vi "Game Engine.vi"(6 "UI Refs":T1, 8 "XY":cluster{"Horizontal":dbl, "Vertical":dbl}, 10 "Dashboard":T2[](array[typedef]), 11 "SquareBattle in":refnum<class "SquareBattle Arena.lvclass">) -> ()   [LabVIEW 2014, in "SquareBattle Arena.lvlib" / "SquareBattle Arena.lvclass"]
uses:
  SquareBattle Arena.lvclass
  Dashboard.ctl
  UI Refs.ctl
  Runner Cluster.ctl
  Square/Square.lvclass
  SquareBattle Arena.lvclass/SquareBattle Arena.ctl
  Action Enum.ctl
  Square/Square.lvclass/Square.ctl
  Endigit Library/Endigit.lvlib
panel:
  out "Penalty":i32(graph)
  out "Total Runners":i32
  out "Elapsed Time":u32
  # "NOTICE - YOU MUST NOT REMOVE THIS NOTICE. PER THE FOLLOWING LICENSE, YOU MAY REPRODUCE THIS SOFTWARE PROVIDED YOU FOLLOW THE TERMS\nOF THE LICENSE.\n\n---BEGIN BSD LICENSE (http://opensource.org/licenses/BSD-2-Clause)---\nCopyright (c) 2015, Endigit, Inc. <robert@endigit.com>\nAll rights reserved.\n\nRedistribution and use in source and binary forms, with or without modification, are permitted provided that the following conditions are met:\n\n1. Redistributions of source code must retain the above copyright notice, this list of conditions and the following disclaimer.\n\n2. Redistributions in binary form must reproduce the above copyright notice, this list of conditions and the following disclaimer in the documentation and/or other \nmaterials provided with the distribution.\n\nTHIS SOFTWARE IS PROVIDED BY THE COPYRIGHT HOLDERS AND CONTRIBUTORS \"AS IS\" AND ANY EXPRESS OR IMPLIED WARRANTIES, INCLUDING, BUT NOT \nLIMITED TO, THE IMPLIED WARRANTIES OF MERCHANTABILITY AND FITNESS FOR A PARTICULAR PURPOSE ARE DISCLAIMED. IN NO EVENT SHALL THE COPYRIGHT \nHOLDER OR CONTRIBUTORS BE LIABLE FOR ANY DIRECT, INDIRECT, INCIDENTAL, SPECIAL, EXEMPLARY, OR CONSEQUENTIAL DAMAGES (INCLUDING, BUT NOT \nLIMITED TO, PROCUREMENT OF SUBSTITUTE GOODS OR SERVICES; LOSS OF USE, DATA, OR PROFITS; OR BUSINESS INTERRUPTION) HOWEVER CAUSED AND ON \nANY THEORY OF LIABILITY, WHETHER IN CONTRACT, STRICT LIABILITY, OR TORT (INCLUDING NEGLIGENCE OR OTHERWISE) ARISING IN ANY WAY OUT OF THE USE \nOF THIS SOFTWARE, EVEN IF ADVISED OF THE POSSIBILITY OF SUCH DAMAGE.\n---END BSD LICENSE---"
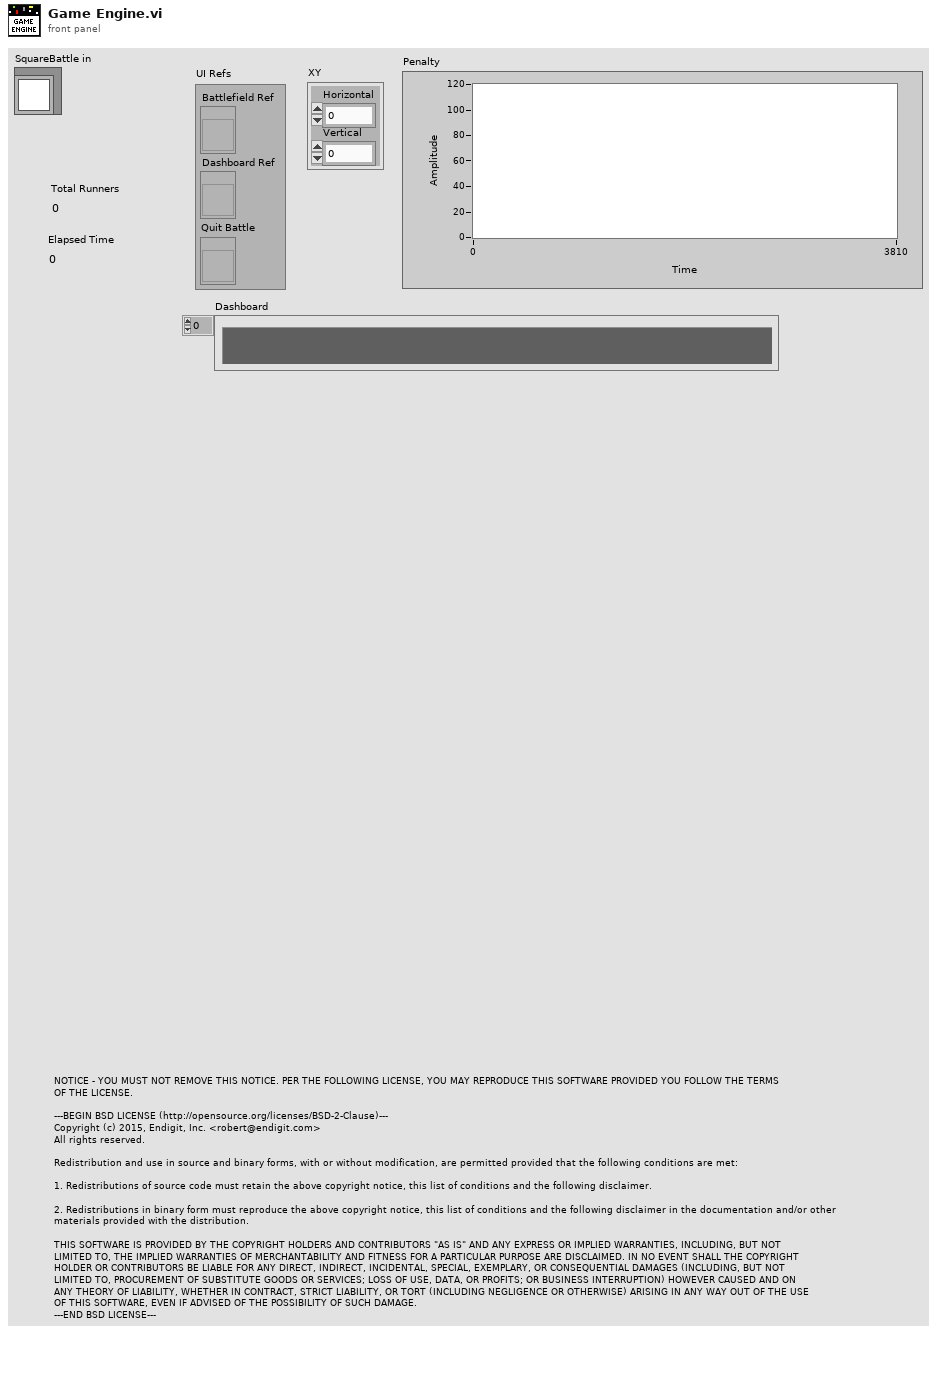
[diagram p1: front panel]
types:
  T1 = typedef "SquareBattle Arena.lvlib/SquareBattle Arena.lvclass/UI Refs.ctl" = cluster{"Battlefield Ref":refnum<vi>, "Dashboard Ref":refnum<vi>, "Quit Battle":refnum<vi>}
  T2 = typedef "SquareBattle Arena.lvlib/SquareBattle Arena.lvclass/Dashboard.ctl" = cluster{"Color":u32, "Player":string, "Status":string}
  T3 = typedef "SquareBattle Arena.lvlib/SquareBattle Arena.lvclass/Runner Cluster.ctl" = cluster{"Attacked?":bool, "DVR":refnum<data-value>, "Team":i32, "Player":i32, "Next Turn":i32, "Penalty":i32}
  T4 = typedef "SquareBattle Arena.lvlib/SquareBattle Arena.lvclass/Action Enum.ctl" = enum16{"Wait", "Move", "Attack", "Replicate"}
  T5 = typedef "SquareBattle Arena.lvlib/SquareBattle Arena.lvclass/Direction Enum.ctl" = enum16{"NW", "N", "NE", "E", "SE", "S", "SW", "W"}
  T6 = cluster{"Cluster":T3, i32, i32, "Action":T4, "Direction":T5, "Replicated":refnum<class "Square.lvclass">}
  T7 = typedef "SquareBattle Arena.lvlib/SquareBattle Arena.lvclass/Player Info.ctl" = cluster{"Name":string, "Color Box":u32, "Gloat Phrase":string}
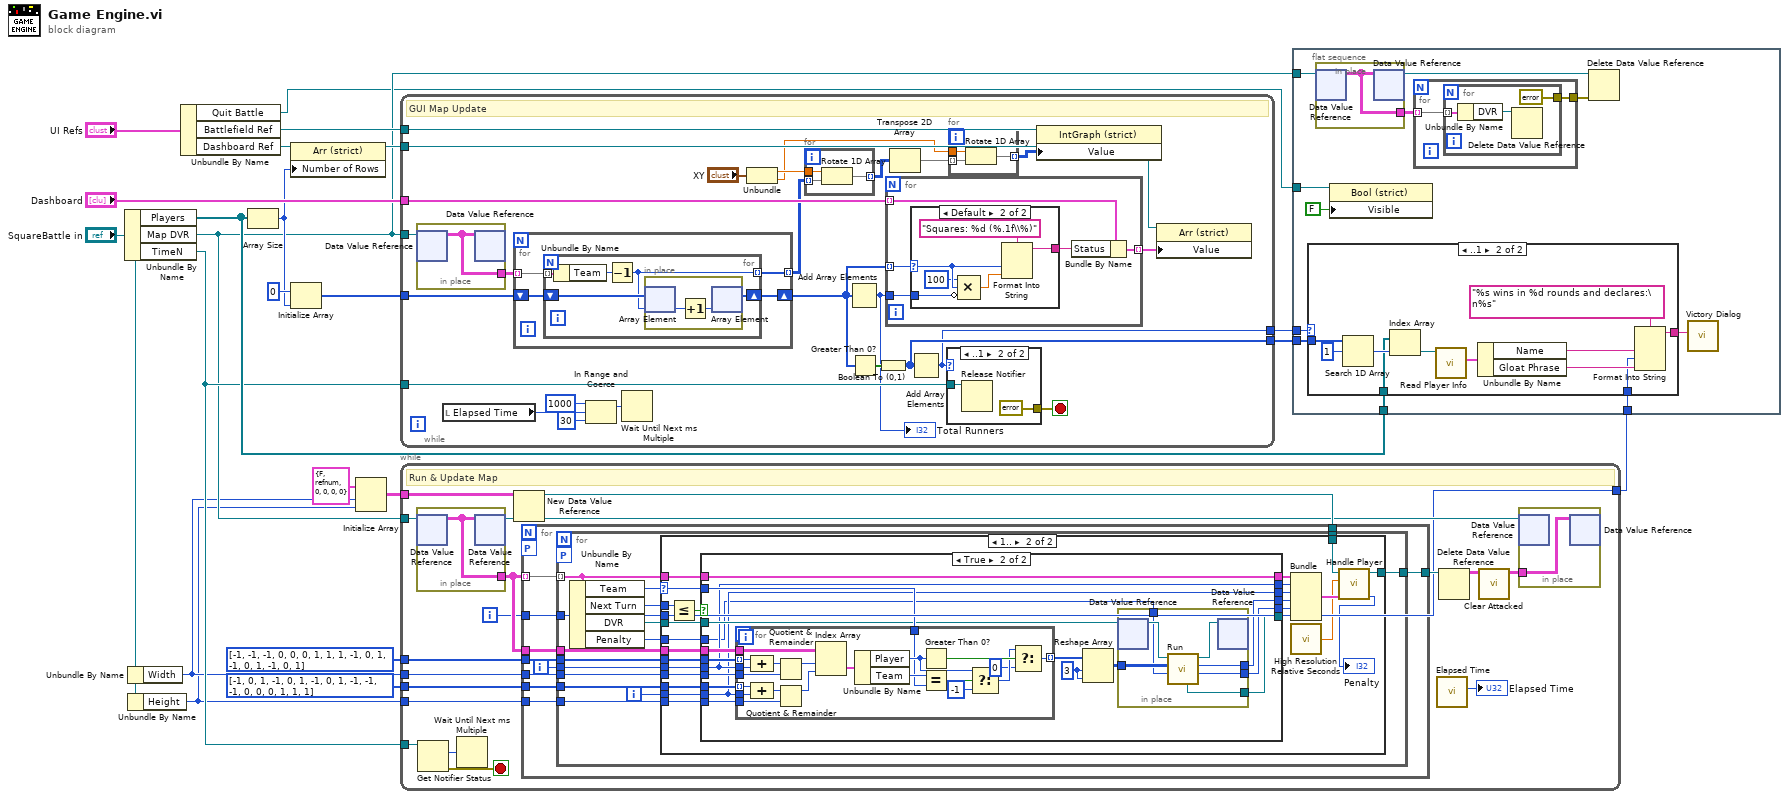
[diagram p0: block diagram]
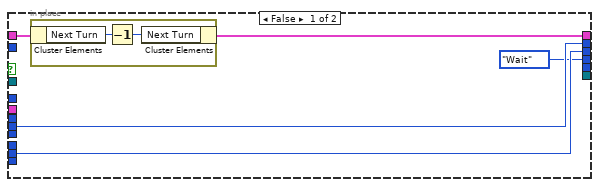
[diagram p3: hidden frame]
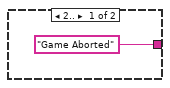
[diagram p4: hidden frame]
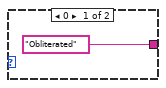
[diagram p5: hidden frame]
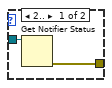
[diagram p6: hidden frame]
diagram:
  n1 = Unbundle By Name("SquareBattle in") -> ("Players"=w12:refnum<class "Square.lvclass">[], "Map DVR"=w10:refnum<data-value>, "TimeN"=w11:refnum<notifier>)
  n2 = Unbundle By Name("SquareBattle in") -> ("Width"=w7:i32)
  n3 = Unbundle By Name("SquareBattle in") -> ("Height"=w6:i32)
  n4 = Unbundle By Name("UI Refs") -> ("Quit Battle"=w4:refnum<vi>, "Battlefield Ref"=w20:refnum<vi>, "Dashboard Ref"=w17:refnum<vi>)
  n5 = Array Size(array=w12) -> (size(s)=w14:i32)
  n6 = property on="Property Node" class="Arr (strict)"(reference=w17, "Number of Rows"=w14) -> (reference out=w16:refnum<vi>)  [unwired: 1 in, 1 out]
  n7 = Initialize Array(0 ("element"), w14) -> (w13:i32[])
  n8 = Initialize Array(T3 {"Attacked?"=FALSE, "DVR"=refnum, "Team"=0, "Player"=0, "Next Turn"=0, "Penalty"=0} ("Cluster"), w7, w6) -> (w5:T3[][])
  n9 = while {
    tunnel: "Dashboard" -> [w45]
    tunnel: w16 -> [w42]
    tunnel: w20 -> [w26]
    tunnel: [w34] -> w19
    tunnel: [w33] -> w18
    tunnel: w10 -> [w36]
    tunnel: w11 -> [w38]
    tunnel: w13 -> [w37]
    stop <- w46 stop-if-true
    # "GUI Map Update"
    n10 = in-place {
      in-place-border: [w65] -> w35
      n11 = in-place-dvr #1(w36) -> (w65:T3[][])  [unwired: 1 out]
      n12 = in-place-dvr #1(w65) -> ()  [unwired: 2 out]
    }
    n13 = local read "Elapsed Time"() -> (w31:u32)
    n14 = for {
      tunnel: w35 -> [w55] mode=indexing
      tunnel: [w54] -> w30 mode=indexing
      shift-right: [w57] -> w44
      shift-left: w37 -> [w56]
      n15 = for {
        shift-right: [w62] -> w57
        shift-left: w56 -> [w61]
        tunnel: w55 -> [w60] mode=indexing
        tunnel: [w58] -> w54 mode=indexing
        n16 = Unbundle By Name(w60) -> ("Team"=w59:i32)
        n17 = Decrement(x=w59) -> (x-1=w58:i32)
        n18 = in-place {
          n19 = in-place-array #2(w61, w58) -> (w64:i32)
          n20 = Increment(x=w64) -> (x+1=w63:i32)
          n21 = in-place-array #2(w63) -> (w62:i32[])  [unwired: 1 out]
        }
      }
    }
    n22 = In Range and Coerce(upper limit=u32 1000 ("millisecond multiple"), x=w31, lower limit=u32 30) -> (coerced(x)=w41:u32)  [unwired: 1 out]
    n23 = Wait Until Next ms Multiple(millisecond multiple=w41) -> ()  [unwired: 1 out]
    n24 = Unbundle("XY") -> ("Horizontal"=w24:dbl, "Vertical"=w23:dbl)
    n25 = for {
      tunnel: w30 -> [w53] mode=indexing
      tunnel: [w52] -> w29 mode=indexing
      tunnel: w24 -> [w51]
      n26 = Rotate 1D Array(1:w53, 2:w51) -> (0:w52:i32[])
    }
    n27 = Add Array Elements(numeric array=w44) -> (sum=w32:i32)
    "Total Runners" <- w32
    n28 = Greater Than 0?(x=w44) -> (x > 0?=w47:bool[])
    n29 = Boolean To (0,1)(Boolean=w47) -> (0, 1=w34:i16[])
    n30 = for {
      tunnel: w45 -> [w70] mode=indexing
      tunnel: [w69] -> w43 mode=indexing
      tunnel: w44 -> [w66] mode=indexing
      tunnel: w32 -> [w67]
      n31 = case shown="Default" w66 {
        selector: w66 -> [_ w74]
        tunnel: ["Obliterated" w76] -> w68
        tunnel: w67 -> [_ w73]
        frame 0 {
        }
        frame Default {
          n32 = Compound Arithmetic op=MULTIPLY(100 ("value"), w74, invert w73) -> (w75:dbl)
          n33 = Format Into String(format string="Squares: %d (%.1f\\%)", w74, w75) -> (resulting string=w76:string)  [unwired: 2 in, 1 out]
        }
      }
      n34 = Bundle By Name(cluster=w70, "Status"=w68) -> (w69:T2)
    }
    n35 = Transpose 2D Array(2D array=w29) -> (transposed array=w28:i32[][])
    n36 = Add Array Elements(numeric array=w34) -> (sum=w33:i16)
    n37 = case shown="..1" w33 {
      tunnel: w38 -> [w79 w81]
      tunnel: [w78 errorcluster {"status"=TRUE, "code"=0, "source"=""} ("error out")] -> w46
      frame 2.. {
        n38 = Get Notifier Status(notifier=w79) -> (error out=w78:errorcluster)  [unwired: 1 in, 4 out]
      }
      frame ..1 {
        n39 = Release Notifier(notifier=w81) -> ()  [unwired: 2 in, 3 out]
      }
    }
    n40 = for {
      tunnel: w28 -> [w50] mode=indexing
      tunnel: [w49] -> w27 mode=indexing
      tunnel: w23 -> [w48]
      n41 = Rotate 1D Array(1:w50, 2:w48) -> (0:w49:i32[])
    }
    n42 = property on="Property Node" class="IntGraph (strict)"(reference=w26, "Value"=w27) -> ()  [unwired: 1 in, 2 out]
    n43 = property on="Property Node" class="Arr (strict)"(reference=w42, "Value"=w43) -> ()  [unwired: 1 in, 2 out]
  }
  n44 = while {
    tunnel: w11 -> [w97]
    tunnel: w10 -> [w95]
    tunnel: i32[] [-1, -1, -1, 0, 0, 0, 1, 1, 1, -1, 0, 1, -1, 0, 1, -1, 0, 1] -> [w93]
    tunnel: w7 -> [w92]
    tunnel: i32[] [-1, 0, 1, -1, 0, 1, -1, 0, 1, -1, -1, -1, 0, 0, 0, 1, 1, 1] -> [w90]
    tunnel: w6 -> [w91]
    tunnel: w5 -> [w89]
    tunnel: [w82] -> w1
    i -> [w82]
    stop <- w96 stop-if-true
    # "Run & Update Map"
    n45 = in-place {
      in-place-border: [w203] -> w94
      n46 = in-place-dvr #3(w95) -> (w203:T3[][])  [unwired: 1 out]
      n47 = in-place-dvr #3(w203) -> (w86:refnum<data-value>)  [unwired: 1 out]
    }
    n48 = Get Notifier Status(notifier=w97) -> (current notification=w98:u32, error out=w96:errorcluster)  [unwired: 1 in, 3 out]
    n49 = Wait Until Next ms Multiple(millisecond multiple=w98) -> ()  [unwired: 1 out]
    n50 = New Data Value Reference(data value=w89) -> (data value reference=w88:refnum<data-value>)  [unwired: 1 in, 1 out]
    n51 = for {
      tunnel: w94 -> [w109] mode=indexing
      tunnel: w82 -> [w108]
      tunnel: w94 -> [w107]
      tunnel: w93 -> [w106]
      tunnel: w92 -> [w104]
      tunnel: w90 -> [w102]
      tunnel: w91 -> [w103]
      tunnel: w88 -> [w101]
      tunnel: [w100] -> w87
      workers-P: _ -> [_]
      i -> [w105]
      n52 = for {
        tunnel: w109 -> [w115] mode=indexing
        tunnel: w108 -> [w114]
        tunnel: w107 -> [w124]
        tunnel: w106 -> [w123]
        tunnel: w105 -> [w122]
        tunnel: w104 -> [w121]
        tunnel: w102 -> [w119]
        tunnel: w103 -> [w120]
        workers-P: _ -> [_]
        tunnel: w101 -> [w112]
        tunnel: [w111] -> w100
        i -> [w118]
        n53 = Unbundle By Name(w115) -> ("Team"=w116:i32, "Next Turn"=w113:i32, "DVR"=w117:refnum<data-value>, "Penalty"=w110:i32)
        n54 = case shown="1.." w116 {
          selector: w116 -> [_ w145]
          tunnel: w124 -> [_ w150]
          tunnel: w123 -> [_ w149]
          tunnel: w122 -> [_ w142]
          tunnel: w121 -> [_ w148]
          tunnel: w119 -> [_ w146]
          tunnel: w118 -> [_ w141]
          tunnel: w120 -> [_ w147]
          tunnel: w117 -> [_ w144]
          tunnel: w115 -> [_ w143]
          tunnel: w114 -> [_ w140]
          tunnel: w113 -> [_ w139]
          tunnel: w112 -> [w125 w130]
          tunnel: [w125 w129] -> w111
          tunnel: w110 -> [_ w126]
          frame ..0 {
          }
          frame 1.. {
            n55 = Less Or Equal?(x=w139, y=w140) -> (x <= y?=w138:bool)
            n56 = case shown="True" w138 {
              tunnel: w150 -> [_ w174]
              tunnel: w149 -> [_ w173]
              tunnel: w148 -> [_ w172]
              tunnel: w147 -> [_ w171]
              tunnel: w146 -> [_ w170]
              tunnel: w145 -> [_ w167]
              tunnel: w144 -> [_ w165]
              tunnel: w143 -> [w152 w164]
              tunnel: w142 -> [w155 w163]
              tunnel: w141 -> [w154 w162]
              tunnel: [w151 w164] -> w137
              tunnel: [w155 w163] -> w136
              tunnel: [w154 w162] -> w135
              tunnel: [Action_Enum."Wait" ("Action") w161] -> w134
              tunnel: [_ w160] -> w133
              tunnel: [_ w159] -> w132
              tunnel: w126 -> [_ w158]
              frame False {
                n57 = in-place {
                  n58 = in-place-cluster #4(w152) -> ("Next Turn"=w157:i32)
                  n59 = Decrement(x=w157) -> (x-1=w156:i32)
                  n60 = in-place-cluster #4("Next Turn"=w156) -> (w151:T3)
                }
              }
              frame True {
                w168 = 3 ("dimension size")
                n61 = for {
                  tunnel: w174 -> [w202]
                  tunnel: w173 -> [w201] mode=indexing
                  tunnel: w163 -> [w200]
                  tunnel: w172 -> [w198]
                  tunnel: w170 -> [w194] mode=indexing
                  tunnel: w162 -> [w195]
                  tunnel: w171 -> [w196]
                  tunnel: [w183] -> w169 mode=indexing
                  tunnel: w167 -> [w182]
                  n62 = Compound Arithmetic op=ADD(w201, w200) -> (w199:i32)
                  n63 = Compound Arithmetic op=ADD(w194, w195) -> (w193:i32)
                  n64 = Quotient & Remainder(x=w199, y=w198) -> (x-y*floor(x/y)=w197:i32)  [unwired: 1 out]
                  n65 = Quotient & Remainder(x=w193, y=w196) -> (x-y*floor(x/y)=w192:i32)  [unwired: 1 out]
                  n66 = Index Array(array=w202, index (row)=w197, index (col)=w192) -> (element=w191:T3)
                  n67 = Unbundle By Name(w191) -> ("Player"=w188:i32, "Team"=w190:i32)
                  n68 = Greater Than 0?(x=w188) -> (x > 0?=w187:bool)
                  n69 = Equal?(x=w190, y=w182) -> (x = y?=w189:bool)
                  n70 = Select(t=w188, s=w189, f=-1) -> (s? t:f=w185:i32)
                  n71 = Select(t=w185, s=w187, f=0) -> (s? t:f=w183:i32)
                }
                n72 = Reshape Array(w169, w168, w168) -> (w166:i32[][])
                n73 = in-place {
                  in-place-border: w166 -> [w179]
                  in-place-border: [w178] -> w161
                  in-place-border: [w177] -> w160
                  in-place-border: [w176] -> w159
                  in-place-border: w158 -> [w175]
                  n74 = in-place-dvr #5(w165) -> (w181:refnum<class "Square.lvclass">)  [unwired: 1 out]
                  n75 = call-dynamic "Run.vi"("Penalty"=w175, "Maze (0: Empty, -1: Enemy. 1: Teammate"=w179, "Runner in"=w181) -> ("Direction"=w177:T5, "Action"=w178:T4, "Runner out"=w180:refnum<class "Square.lvclass">, "Replicated"=w176:refnum<class "Square.lvclass">)  [unwired: 4 in, 1 out]
                  n76 = in-place-dvr #5(w180) -> ()  [unwired: 2 out]
                }
              }
            }
            n77 = Bundle("Cluster"=w137, w136, w135, "Action"=w134, "Direction"=w133, "Replicated"=w132) -> (w131:T6)  [unwired: 1 in]
            n78 = call <vilib>:"High Resolution Relative Seconds.vi"() -> ("relative seconds"=w128:dbl)
            n79 = call "Handle Player.vi"("Move Info"=w131, "Relative Seconds"=w128, "Temp DVR"=w130) -> ("Penalty"=→"Penalty":i32, "Temp DVR"=w129:refnum<data-value>)  [unwired: 7 in]
          }
        }
      }
    }
    n80 = call "Elapsed Time.vi"() -> ("Elapsed Time"=→"Elapsed Time":u32)  [unwired: 11 in]
    n81 = Delete Data Value Reference(data value reference=w87) -> (data value=w84:T3[][])  [unwired: 1 in, 1 out]
    n82 = call "Clear Attacked.vi"("Array in"=w84) -> ("Array out"=w83:T3[][])  [unwired: 10 in]
    n83 = in-place {
      in-place-border: w83 -> [w99]
      n84 = in-place-dvr #6(w86) -> ()  [unwired: 2 out]
      n85 = in-place-dvr #6(w99) -> ()  [unwired: 2 out]
    }
  }
  n86 = flat-sequence {
    tunnel: w19 -> [w214]
    tunnel: w18 -> [w213]
    tunnel: w12 -> [w212]
    tunnel: w10 -> [w211]
    tunnel: w4 -> [w207]
    tunnel: w1 -> [w205]
    frame #0 {
      n87 = case shown="..1" w213 {
        tunnel: ["Game Aborted" w231] -> w204
        tunnel: w214 -> [_ w230]
        tunnel: w212 -> [_ w224]
        tunnel: w205 -> [_ w222]
        frame 2.. {
        }
        frame ..1 {
          n88 = Search 1D Array(1D array=w230, element=i16 1) -> (index of element=w228:i32)  [unwired: 1 in]
          n89 = Index Array(array=w224, index=w228) -> (element=w227:refnum<class "Square.lvclass">)
          n90 = call "Read Player Info.vi"("Runner in"=w227) -> ("Player Info"=w226:T7)  [unwired: 8 in, 2 out]
          n91 = Unbundle By Name(w226) -> ("Name"=w225:string, "Gloat Phrase"=w223:string)
          n92 = Format Into String(format string="%s wins in %d rounds and declares:\n%s", w225, w222, w223) -> (resulting string=w231:string)  [unwired: 2 in, 1 out]
        }
      }
      n93 = in-place {
        in-place-border: [w220] -> w210
        n94 = in-place-dvr #7(w211) -> (w220:T3[][])  [unwired: 1 out]
        n95 = in-place-dvr #7(w220) -> (w209:refnum<data-value>)  [unwired: 1 out]
      }
      n96 = property on="Property Node" class="Bool (strict)"(reference=w207, "Visible"=FALSE) -> ()  [unwired: 1 in, 2 out]
      n97 = for {
        tunnel: w210 -> [w216] mode=indexing
        tunnel: [w215] -> w208
        n98 = for {
          tunnel: w216 -> [w218] mode=indexing
          tunnel: [errorcluster {"status"=FALSE, "code"=0, "source"=""} ("error out")] -> w215
          n99 = Unbundle By Name(w218) -> ("DVR"=w219:refnum<data-value>)
          n100 = Delete Data Value Reference(data value reference=w219) -> ()  [unwired: 1 in, 2 out]
        }
      }
      n101 = Delete Data Value Reference(data value reference=w209, error in=w208) -> ()  [unwired: 2 out]
      n102 = call "Victory Dialog.vi"("Victory Phrase"=w204) -> ()  [unwired: 10 in, 1 out]
    }
  }
